vi "Set IConfiguration.vi"(8 "error in":errorcluster, 10 "IConfiguration":refnum<class "IConfiguration.lvclass">, 11 "NEO480 in":refnum<class "Virtual NEO480.lvclass">) -> (0 "error out":errorcluster, 3 "NEO480 out":refnum<class "Virtual NEO480.lvclass">)   [LabVIEW 2024, in "Virtual NEO480.lvclass"]
uses:
  Virtual NEO480.lvclass
  Source/Interfaces/IConfiguration/IConfiguration.lvclass
  Virtual NEO480.lvclass/Virtual NEO480.ctl
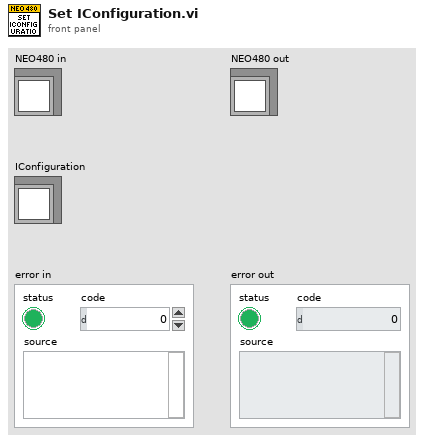
[diagram p1: front panel]
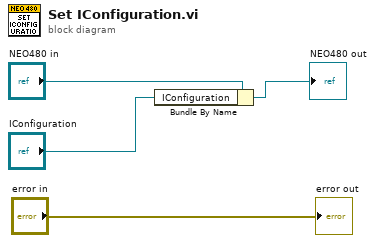
[diagram p0: block diagram]
diagram:
  n1 = Bundle By Name(cluster="NEO480 in", "IConfiguration"="IConfiguration") -> (→"NEO480 out":refnum<class "Virtual NEO480.lvclass">)
  "error out" <- "error in"
